vi "Video Stuff v11.vi"() -> ()   [LabVIEW 2009]
uses:
  <vilib>/userDefined/High Color/IMAQdx.ctl
  <vilib>/vision/NI_Vision_Development_Module.lvlib
  <vilib>/vision/driver/NI_Vision_Acquisition_Software.lvlib
panel:
  in  "Tab Control":enum32{"RGB", "RGB Adaptive", "Raphael", "Dan"}(tab)
  in  "Red Range":cluster{"Lower value":i32, "Upper value":i32}={"Lower value"=33, "Upper value"=255}
  in  "Green Range":cluster{"Lower value":i32, "Upper value":i32}={"Lower value"=0, "Upper value"=255}
  in  "Blue Range":cluster{"Lower value":i32, "Upper value":i32}={"Lower value"=0, "Upper value"=255}
  in  "Blue Scalar":sgl=3.3000002
  in  "Green Scalar":sgl=3.0
  in  "Red Scalar":sgl=4.0
  in  "Threshold Limits":cluster{"Lower value":sgl, "Upper value":sgl}={"Lower value"=0.0, "Upper value"=255.0} {"Upper value" format="%.2f"; "Lower value" format="%.2f"}
  out "Threshold Range Out":cluster{"Lower value":sgl, "Upper value":sgl}={"Lower value"=139.0, "Upper value"=255.0} {"Upper value" format="%.2f"; "Lower value" format="%.2f"}
  out "Number of Particles":i32=3
  in  "Selection Values":T2(array[cluster])=[{"Measurement Parameter"=35, "Range Lower Value"=100.0, "Range Upper Value"=10000.0, "Range"=FALSE, "Measurement Type"=FALSE}] {"Measurement Parameter" items=["Center of Mass X", "Center of Mass Y", "First Pixel X", "First Pixel Y", "Bounding Rect Left", "Bounding Rect Top", "Bounding Rect Right", "Bounding Rect Bottom", "Max Feret Diameter Start X", "Max Feret Diameter Start Y", "Max Feret Diameter End X", "Max Feret Diameter End Y", "Max Horiz. Segment Length Left", "Max Horiz. Segment Length Right", "Max Horiz. Segment Length Row", "-", "Bounding Rect Width", "Bounding Rect Height", "Bounding Rect Diagonal", "Perimeter", "Convex Hull Perimeter", "Holes' Perimeter", "Max Feret Diameter", "Equivalent Ellipse Major Axis", "Equivalent Ellipse Minor Axis", "Equivalent Ellipse Minor Axis (Feret)", "Equivalent Rect Long Side", "Equivalent Rect Short Side", "Equivalent Rect Diagonal", "Equivalent Rect Short Side (Feret)", "Average Horiz. Segment Length", "Average Vert. Segment Length", "Hydraulic Radius", "Waddel Disk Diameter", "-", "Area", "Holes' Area", "Particle & Holes' Area", "Convex Hull Area", "Image Area", "-", "Number of Holes", "Number of Horiz. Segments", "Number of Vert. Segments", "-", "Orientation", "Max Feret Diameter Orientation", "-", "% Area/Image Area", "% Area/(Particle & Holes' Area)", "Ratio of Equivalent Ellipse Axes", "Ratio of Equivalent Rect Sides", "-", "Elongation Factor", "Compactness Factor", "Heywood Circularity Factor", "Type Factor", "-", "Sum X", "Sum Y", "Sum XX", "Sum XY", "Sum YY", "Sum XXX", "Sum XXY", "Sum XYY", "Sum YYY", "-", "Moment of Inertia XX", "Moment of Inertia XY", "Moment of Inertia YY", "Moment of Inertia XXX", "Moment of Inertia XXY", "Moment of Inertia XYY", "Moment of Inertia YYY", "Norm. Moment of Inertia XX", "Norm. Moment of Inertia XY", "Norm. Moment of Inertia YY", "Norm. Moment of Inertia XXX", "Norm. Moment of Inertia XXY", "Norm. Moment of Inertia XYY", "Norm. Moment of Inertia YYY", "Hu Moment 1", "Hu Moment 2", "Hu Moment 3", "Hu Moment 4", "Hu Moment 5", "Hu Moment 6", "Hu Moment 7"]}
  in  "Filter Select":T3(radio)
  in  "bin 1    bin 2":bool
  in  "Select Filter":enum16{"RGB", "RGB Adaptive", "Raphael", "Dan"}(ring)=enum."RGB Adaptive"
  out "Live Video 2":T4(plugin-control)
  in  "Y Min":i32=2
  in  "Y Max":i32=13
  in  "X min":i32=2
  in  "X max":i32=15
  in  "Desired X Resolution":i32=640
  in  "LineFilterSelect":bool=TRUE
  out "Hough Intensity Graph":i32[][](graph)
  out "Angle 2":i32=25
  out "X Intercept 2":i32=-500
  in  "Hough Skip":i32=1
  out "Waypoint":cluster{i32, i32}={132, 5}
  in  "WP_DisplaySize/2":i32
  out "Filter Binary 2":T4(plugin-control)
  in  "Offset scale":dbl=1.51
  in  "Y":i32=1741
  in  "X":i32=777
  out "Real World Coordinates":cluster{"X":sgl, "Y":sgl}={"X"=76.907585, "Y"=411.85178} {"Y" format="%.2f"; "X" format="%.2f"}
  in  "Interpolation Type":u32(ring)=1 items=["Zero Order", "Bi-Linear", "Quadratic", "Cubic Spline"]
  in  "X Resolution":i32=640
  in  "Numeric":i32=21
  out "Occupancy Grid Square Size":dbl=5.022463525777591
  in  "LIDAR/Wheel Position Offset (in.)":dbl=60.0
  out "\"Obstickles\" y":dbl[](array[numeric])=[303.34102199907545, 303.34102199907545, 303.34102199907545, 303.34102199907545, 303.34102199907545, 295.75710207515135, 295.75710207515135, 295.75710207515135, 295.75710207515135, 295.75710207515135, 295.75710207515135, 295.75710207515135, 295.75710207515135, 295.75710207515135, 295.75710207515135, 295.75710207515135, 295.75710207515135, 295.75710207515135, 295.75710207515135, 288.1731821512272, 288.1731821512272, 288.1731821512272, 288.1731821512272, 288.1731821512272, 288.1731821512272, 288.1731821512272, 288.1731821512272, 288.1731821512272, 288.1731821512272, 288.1731821512272, 288.1731821512272, 288.1731821512272, 288.1731821512272, 288.1731821512272, 280.58926222730304, 280.58926222730304, 280.58926222730304, 280.58926222730304, 280.58926222730304, 280.58926222730304, 280.58926222730304, 280.58926222730304, 280.58926222730304, 280.58926222730304, 280.58926222730304, 280.58926222730304, 280.58926222730304, 280.58926222730304, 280.58926222730304, 280.58926222730304, 273.0053423033788, 273.0053423033788, 273.0053423033788, 273.0053423033788, 273.0053423033788, 273.0053423033788, 273.0053423033788, 273.0053423033788, 273.0053423033788, 273.0053423033788, 273.0053423033788, 273.0053423033788, 273.0053423033788, 273.0053423033788, 273.0053423033788, 273.0053423033788, 273.0053423033788, 265.4214223794547, 265.4214223794547, 265.4214223794547, 265.4214223794547, 265.4214223794547, 265.4214223794547, 265.4214223794547, 265.4214223794547, 265.4214223794547, 265.4214223794547, 265.4214223794547, 265.4214223794547, 265.4214223794547, 257.8375024555305, 257.8375024555305, 257.8375024555305, 257.8375024555305, 257.8375024555305, 257.8375024555305, 257.8375024555305, 257.8375024555305, 257.8375024555305, 257.8375024555305, 250.25358253160636, 250.25358253160636, 250.25358253160636, 250.25358253160636, 250.25358253160636, 250.25358253160636, 250.25358253160636, 250.25358253160636, 250.25358253160636, 250.25358253160636, 250.25358253160636, 242.6696626076822, 242.6696626076822, 242.6696626076822, 242.6696626076822, 242.6696626076822, 242.6696626076822, 242.6696626076822, 242.6696626076822, 235.085742683758, 235.085742683758, 235.085742683758, 235.085742683758, 235.085742683758, 235.085742683758, 227.50182275983389, 227.50182275983389, 227.50182275983389, 219.9179028359097, 219.9179028359097, 219.9179028359097, 219.9179028359097, 212.33398291198554, 212.33398291198554, 212.33398291198554, 212.33398291198554, 212.33398291198554, 212.33398291198554, 212.33398291198554, 212.33398291198554, 204.7500629880614, 204.7500629880614, 204.7500629880614, 204.7500629880614, 204.7500629880614, 189.58222314021305, 181.9983032162889, 174.41438329236473, 174.41438329236473, 166.83046336844058, 166.83046336844058, 159.2465434445164, 159.2465434445164, 159.2465434445164, 159.2465434445164, 159.2465434445164, 151.66262352059223, 151.66262352059223, 151.66262352059223, 144.07870359666808, 144.07870359666808, 144.07870359666808, 136.49478367274392, 136.49478367274392, 136.49478367274392, 136.49478367274392, 128.91086374881974, 128.91086374881974, 121.32694382489558, 113.74302390097142, 113.74302390097142, 106.15910397704727, 75.82342428135061]
  out "\"Obstickles\" x":dbl[](array[numeric])=[-83.4231191631658, -75.83919923924164, -68.25527931531747, -60.6713593913933, -53.087439467469146, -83.4231191631658, -75.83919923924164, -68.25527931531747, -60.6713593913933, -53.087439467469146, -30.33567969569665, -22.751759771772488, -15.167839847848326, -7.583919923924163, 0.0, 7.583919923924163, 15.167839847848326, 37.91959961962082, 45.503519543544975, -91.00703908708995, -83.4231191631658, -75.83919923924164, -68.25527931531747, -60.6713593913933, -53.087439467469146, -45.503519543544975, -30.33567969569665, -22.751759771772488, -7.583919923924163, 7.583919923924163, 22.751759771772488, 37.91959961962082, 45.503519543544975, 106.17487893493829, -98.59095901101412, -91.00703908708995, -83.4231191631658, -75.83919923924164, -68.25527931531747, -53.087439467469146, -45.503519543544975, -37.91959961962082, -22.751759771772488, 7.583919923924163, 15.167839847848326, 22.751759771772488, 30.33567969569665, 37.91959961962082, 75.83919923924164, 106.17487893493829, -106.17487893493829, -83.4231191631658, -75.83919923924164, -68.25527931531747, -60.6713593913933, -53.087439467469146, -37.91959961962082, -15.167839847848326, 7.583919923924163, 15.167839847848326, 22.751759771772488, 30.33567969569665, 37.91959961962082, 45.503519543544975, 53.087439467469146, 75.83919923924164, 98.59095901101412, -98.59095901101412, -83.4231191631658, -75.83919923924164, -68.25527931531747, 7.583919923924163, 15.167839847848326, 22.751759771772488, 30.33567969569665, 37.91959961962082, 45.503519543544975, 53.087439467469146, 75.83919923924164, 83.4231191631658, -45.503519543544975, -22.751759771772488, 7.583919923924163, 15.167839847848326, 22.751759771772488, 30.33567969569665, 37.91959961962082, 45.503519543544975, 60.6713593913933, 68.25527931531747, -37.91959961962082, -7.583919923924163, 0.0, 7.583919923924163, 15.167839847848326, 22.751759771772488, 30.33567969569665, 37.91959961962082, 45.503519543544975, 53.087439467469146, 60.6713593913933, -91.00703908708995, 7.583919923924163, 15.167839847848326, 22.751759771772488, 30.33567969569665, 37.91959961962082, 45.503519543544975, 53.087439467469146, -91.00703908708995, -7.583919923924163, 7.583919923924163, 15.167839847848326, 22.751759771772488, 37.91959961962082, -91.00703908708995, 7.583919923924163, 37.91959961962082, -22.751759771772488, 0.0, 22.751759771772488, 30.33567969569665, -15.167839847848326, 0.0, 7.583919923924163, 15.167839847848326, 22.751759771772488, 30.33567969569665, 53.087439467469146, 68.25527931531747, -30.33567969569665, 0.0, 22.751759771772488, 30.33567969569665, 45.503519543544975, 22.751759771772488, 30.33567969569665, 30.33567969569665, 60.6713593913933, -22.751759771772488, 30.33567969569665, -45.503519543544975, -22.751759771772488, 0.0, 30.33567969569665, 37.91959961962082, 22.751759771772488, 37.91959961962082, 45.503519543544975, 22.751759771772488, 45.503519543544975, 53.087439467469146, 0.0, 15.167839847848326, 22.751759771772488, 53.087439467469146, -15.167839847848326, 53.087439467469146, 60.6713593913933, 22.751759771772488, 68.25527931531747, 75.83919923924164, 15.167839847848326]
  out "Small":T4(plugin-control)
  in  "Horizontal Resolution of Small Image":i32=50
  out "Super Filter":T4(plugin-control)
  in  "Color Mode":u16(ring) items=["RGB", "HSL", "HSV", "HSI"]
  in  "stop":bool
  out "Calibrated Image":T4(plugin-control)
  out "Buffer Number":u32=946
  out "Live Video":T4(plugin-control)
  in  "Video Modes":i32(listbox)=20
  in  "Camera Name":T5="cam3"
  in  "Calibration File Path":path=path "C:/Documents and Settings/ekolker/My Documents/OGRE/vision/shoopCal.png"
  out "Top Image":T4(plugin-control) caption="Calibration Template"
  # "Line Width Paramaters"
  # "Indoor\nLower:\n   YUV?\n  150, 180, 20\n   RGB?\n  240, 240, 240"
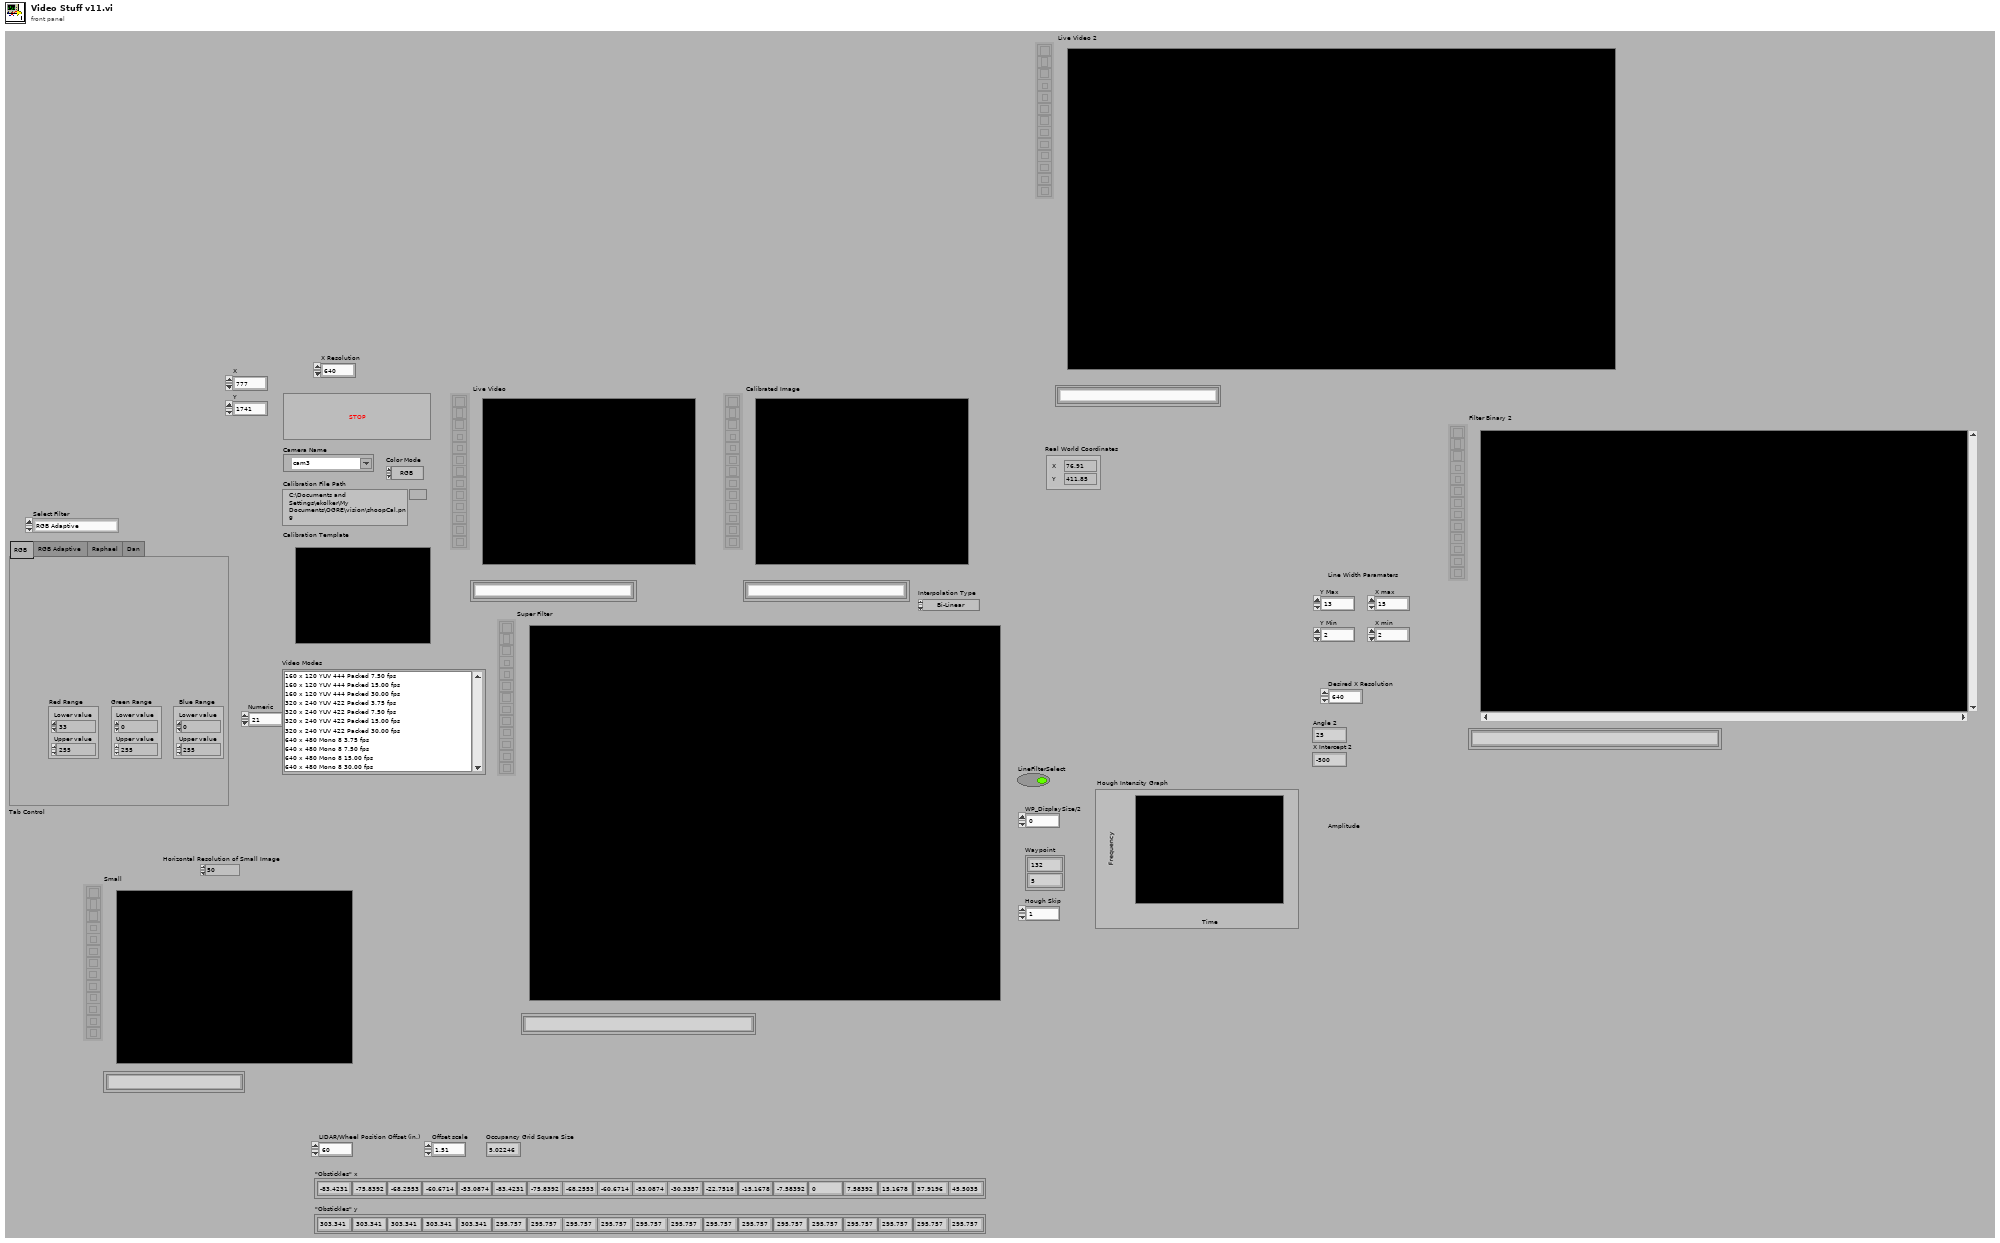
[diagram p1: front panel]
types:
  T1 = typedef "Particle Parameters" = i32
  T2 = cluster{"Measurement Parameter":T1, "Range Lower Value":dbl, "Range Upper Value":dbl, "Range":bool, "Measurement Type":bool}[]
  T3 = enum32{"RGB", "HSL", "RGB Adaptive", "HSL Adaptive", "ANN"}
  T4 = typedef "IMAQ Image.ctl" = refnum<image>
  T5 = typedef "IMAQdx.ctl" = refnum<k21>
  T6 = typedef "Image Type" = u32
  T7 = cluster{"X Step":sgl, "Y Step":sgl, "Unit":u32, "Threshold Range":cluster{"Lower value":sgl, "Upper value":sgl}}
  T8 = cluster{"Distortion":u32, "Corrected Image Scaling":u32, "Corrected Image Learn ROI":u32, "Learn Error Map?":bool, "Learn Correction Table?":bool}
  T9 = cluster{cluster{sgl, sgl}, "Angle Relative to Horizontal (deg)":sgl, "Axis Reference":u32}
  T10 = cluster{"Left":i32, "Top":i32, "Right":i32, "Bottom":i32}
  T11 = cluster{"histogram":u32[], "Minimal Value":sgl, "Maximal Value":sgl, "Starting Value":sgl, "Interval Width":sgl, "Mean Value":sgl, "Standard  Variation":sgl, "Area (pixels)":i32}
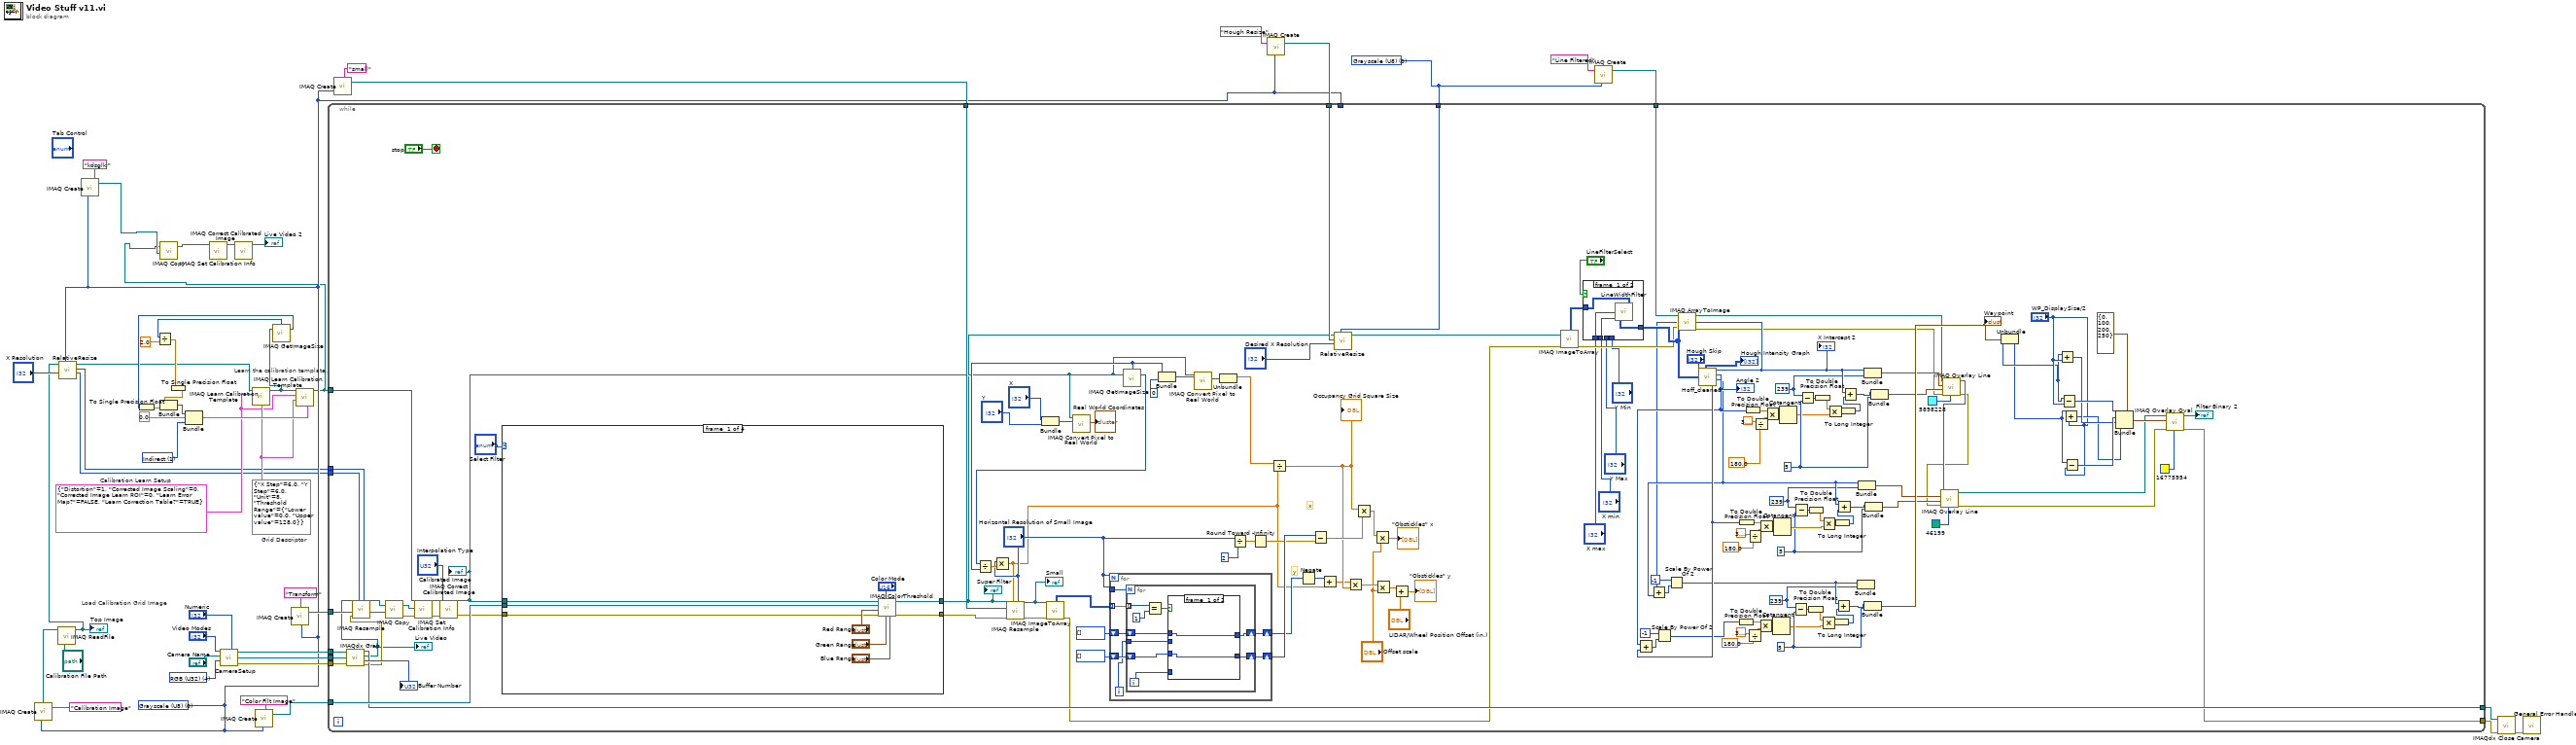
[diagram p0: block diagram]
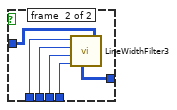
[diagram p2: hidden frame]
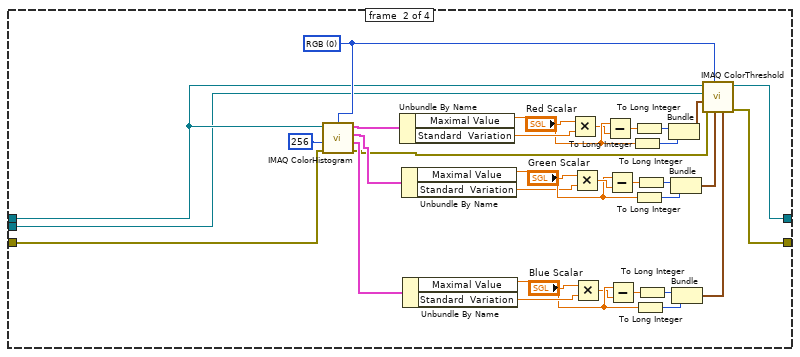
[diagram p3: hidden frame]
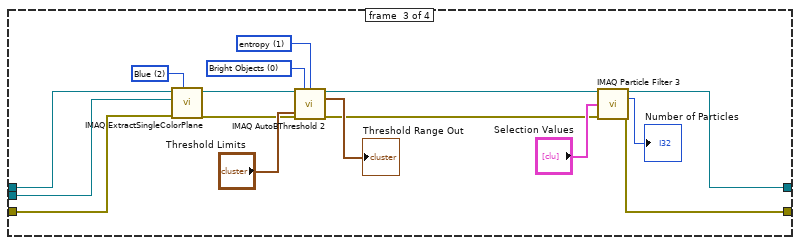
[diagram p4: hidden frame]
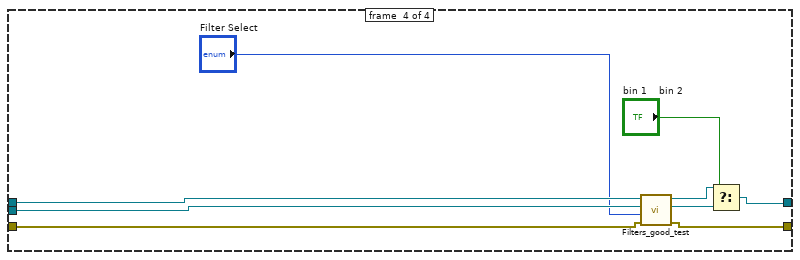
[diagram p5: hidden frame]
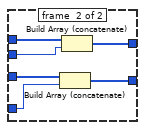
[diagram p6: hidden frame]
diagram:
  w1 = T6 0 items=["Grayscale (U8)", "Grayscale (I16)", "Grayscale (SGL)", "Complex (CSG)", "RGB (U32)", "HSL (U32)", "RGB (U64)", "Grayscale (U16)"] ("Image Type")
  w12 = T6 4 items=["Grayscale (U8)", "Grayscale (I16)", "Grayscale (SGL)", "Complex (CSG)", "RGB (U32)", "HSL (U32)", "RGB (U64)", "Grayscale (U16)"] ("Image Type")
  w31 = u32 1 items=["Direct", "Indirect"] ("Axis Reference")
  w9 = T6 0 items=["Grayscale (U8)", "Grayscale (I16)", "Grayscale (SGL)", "Complex (CSG)", "RGB (U32)", "HSL (U32)", "RGB (U64)", "Grayscale (U16)"] ("Image Type")
  w21 = T7 {"X Step"=6.0, "Y Step"=6.0, "Unit"=8, "Threshold Range"={"Lower value"=0.0, "Upper value"=128.0}}  # Grid Descriptor
  w20 = T8 {"Distortion"=1, "Corrected Image Scaling"=0, "Corrected Image Learn ROI"=0, "Learn Error Map?"=FALSE, "Learn Correction Table?"=TRUE}  # Calibration Learn Setup
  # "Load Calibration Grid Image"
  # "Learn the calibration template."
  n1 = call "IMAQ Create"("Image Name"="Calibration Image", "Image Type"=w9) -> ("New Image"=w39:T4)  [unwired: 2 in, 2 out]
  n2 = call "IMAQ ReadFile"("File Path"="Calibration File Path", "Image"=w39) -> ("Image Out"=w15:T4)  [unwired: 3 in, 6 out]
  "Top Image" <- w15
  n3 = call "RelativeResize.vi"("Image Type"=w9, "Desired X Resolution"="X Resolution", "Image"=w15) -> ("Y Resolution"=w5:i32, "X Resolution"=w4:i32, "Image Dst Out"=w16:T4)  [unwired: 3 in, 1 out]
  n4 = call "IMAQ Create"("Image Name"="kdsglk;", "Image Type"=w9) -> ("New Image"=w3:T4)  [unwired: 2 in, 2 out]
  n5 = call "CameraSetup.vi"("Video Modes"="Video Modes", "Camera Name"="Camera Name", "Image Type"=w12, "Numeric"="Numeric") -> ("Session Out"=w42:T5, "New Image"=w41:T4, "error out"=w40:errorcluster)  [unwired: 2 in]
  n6 = call "IMAQ Learn Calibration Template"("Grid Descriptor"=w21, "Calibration Learn Setup"=w20, "Image"=w16) -> ("Calibrated Image"=w7:T4)  [unwired: 4 in, 4 out]
  n7 = call "IMAQ Create"("Image Name"="Color Filt Image", "Image Type"=w9) -> ("New Image"=w38:T4)  [unwired: 2 in, 2 out]
  n8 = call "IMAQ GetImageSize"("Image"=w7) -> ("Y Resolution"=w25:i32, "X Resolution"=w26:i32)  [unwired: 3 in, 1 out]
  n9 = To Single Precision Float(number=w25) -> (single precision float=w24:sgl)
  n10 = Divide(x=w26, y=2.0) -> (x/y=w23:dbl)
  n11 = To Single Precision Float(number=w23) -> (single precision float=w22:sgl)
  n12 = Bundle(w22, w24) -> (w29:cluster{sgl, sgl})  [unwired: 1 in]
  n13 = Bundle(w29, "Angle Relative to Horizontal (deg)"=sgl 0.0, "Axis Reference"=w31) -> (w28:T9)  [unwired: 1 in]
  n14 = call "IMAQ Create"("Image Name"="Transform", "Image Type"=w9) -> ("New Image"=w43:T4)  [unwired: 2 in, 2 out]
  n15 = call "IMAQ Learn Calibration Template"("Calibration Axis Info"=w28, "Grid Descriptor"=w21, "Calibration Learn Setup"=w20, "Image"=w7) -> ("Calibrated Image"=w2:T4)  [unwired: 3 in, 4 out]
  n16 = call "IMAQ Copy"("Image Dst"=w3, "Image Src"=w2) -> ("Image Dst Out"=w6:T4)  [unwired: 4 in, 1 out]
  n17 = call "IMAQ Set Calibration Info"("Image Src"=w6) -> ("Calibrated Image"=w11:T4)  [unwired: 3 in, 7 out]
  n18 = call "IMAQ Correct Calibrated Image"("Image Src"=w11) -> ("Corrected Image"=→"Live Video 2":T4)  [unwired: 6 in, 4 out]
  n19 = call "IMAQ Create"("Image Name"="small", "Image Type"=w9) -> ("New Image"=w36:T4)  [unwired: 2 in, 2 out]
  n20 = call "IMAQ Create"("Image Name"="Hough Resize", "Image Type"=w9) -> ("New Image"=w13:T4)  [unwired: 2 in, 2 out]
  n21 = call "IMAQ Create"("Image Name"="Line Filtered", "Image Type"=w1) -> ("New Image"=w18:T4)  [unwired: 2 in, 2 out]
  n22 = while {
    tunnel: w2 -> [w165]
    tunnel: w43 -> [w193]
    tunnel: w42 -> [w192]
    tunnel: w41 -> [w191]
    tunnel: w40 -> [w190]
    tunnel: w38 -> [w186]
    tunnel: w36 -> [w184]
    tunnel: [w182] -> w34
    tunnel: [w126] -> w33
    tunnel: w18 -> [w125]
    tunnel: w4 -> [w65]
    tunnel: w5 -> [w64]
    tunnel: w13 -> [w61]
    tunnel: w9 -> [_]
    tunnel: w1 -> [w60]
    stop <- "stop" stop-if-true
    w110 = 5 ("y")
    w109 = 239 ("y")
    w88 = 5 ("y")
    w89 = 239 ("y")
    w77 = 5 ("y")
    w76 = 239 ("y")
    # "y"
    # "x"
    n23 = call <vilib>:"IMAQdx Grab.vi"("error in"=w190, "Image In"=w191, "Session In"=w192) -> ("error out"=w168:errorcluster, "Buffer Number Out"=→"Buffer Number":u32, "Image Out"=w167:T4, "Session Out"=w182:T5)  [unwired: 1 in, 4 out]
    "Live Video" <- w167
    n24 = call "IMAQ Resample"("X Resolution"=w65, "Y Resolution"=w64, "error in (no error)"=w168, "Image Src"=w167) -> ("Image Dst Out"=w166:T4)  [unwired: 6 in, 1 out]
    n25 = call "IMAQ Copy"("Image Dst"=w193, "Image Src"=w166) -> ("error out"=w194:errorcluster, "Image Dst Out"=w197:T4)  [unwired: 4 in]
    n26 = call "IMAQ Set Calibration Info"("error in (no error)"=w194, "Image Dst"=w197, "Image Src"=w165) -> ("error out"=w195:errorcluster, "Calibrated Image"=w196:T4)  [unwired: 1 in, 6 out]
    n27 = call "IMAQ Correct Calibrated Image"("Interpolation Type"="Interpolation Type", "error in (no error)"=w195, "Image Src"=w196) -> ("error out"=w185:errorcluster, "Corrected Image"=w57:T4)  [unwired: 4 in, 3 out]
    "Calibrated Image" <- w57
    n28 = case shown="\"Raphael\"" "Select Filter" {
      tunnel: [w213 w218 w253 w276] -> w189
      tunnel: [w212 w221 w256 w273] -> w56
      tunnel: w186 -> [w211 w222 w262 w274]
      tunnel: w185 -> [w210 w220 w261 w277]
      tunnel: w57 -> [w209 w223 w263 w275]
      frame #0 {
        n29 = call "IMAQ ColorThreshold"("Blue or Luma or Val or Inten Range"="Blue Range", "Green or Sat Range"="Green Range", "Color Mode"="Color Mode", "error in (no error)"=w210, "Red or Hue Range"="Red Range", "Image Dst"=w211, "Image Src"=w209) -> ("error out"=w213:errorcluster, "Image Dst Out"=w212:T4)  [unwired: 3 in]
      }
      frame #1 {
        w251 = u16 0 items=["RGB", "HSL", "HSV", "HSI"] ("Color Mode")
        n30 = call "IMAQ ColorHistogram"("Color Mode"=w251, "Image Src"=w223, "Number of Classes"=256, "error in (no error)"=w220) -> ("Red or Hue or X or L* Histogram Report"=w250:T11, "Green or Sat or Y or a* Histogram Report"=w225:T11, "Blue or Luma or Val or Inten or Z or b* Histogram Report"=w224:T11, "error out"=w219:errorcluster)  [unwired: 2 in]
        n31 = Unbundle By Name(w250) -> ("Maximal Value"=w244:sgl, "Standard  Variation"=w246:sgl)
        n32 = Unbundle By Name(w225) -> ("Maximal Value"=w239:sgl, "Standard  Variation"=w237:sgl)
        n33 = Unbundle By Name(w224) -> ("Maximal Value"=w230:sgl, "Standard  Variation"=w232:sgl)
        n34 = Multiply(x="Red Scalar", y=w246) -> (x*y=w243:sgl)
        n35 = Multiply(x="Green Scalar", y=w237) -> (x*y=w240:sgl)
        n36 = Multiply(x="Blue Scalar", y=w232) -> (x*y=w229:sgl)
        n37 = Subtract(x=w244, y=w243) -> (x-y=w245:sgl)
        n38 = Subtract(x=w239, y=w240) -> (x-y=w238:sgl)
        n39 = Subtract(x=w230, y=w229) -> (x-y=w231:sgl)
        n40 = To Long Integer(number=w244) -> (32bit integer=w247:i32)
        n41 = To Long Integer(number=w245) -> (32bit integer=w248:i32)
        n42 = To Long Integer(number=w239) -> (32bit integer=w236:i32)
        n43 = To Long Integer(number=w230) -> (32bit integer=w233:i32)
        n44 = To Long Integer(number=w238) -> (32bit integer=w235:i32)
        n45 = To Long Integer(number=w231) -> (32bit integer=w234:i32)
        n46 = Bundle(w248, w247) -> (w249:cluster{i32, i32})  [unwired: 1 in]
        n47 = Bundle(w235, w236) -> (w227:cluster{i32, i32})  [unwired: 1 in]
        n48 = Bundle(w234, w233) -> (w226:cluster{i32, i32})  [unwired: 1 in]
        n49 = call "IMAQ ColorThreshold"("Blue or Luma or Val or Inten Range"=w226, "Green or Sat Range"=w227, "Color Mode"=w251, "error in (no error)"=w219, "Red or Hue Range"=w249, "Image Dst"=w222, "Image Src"=w223) -> ("error out"=w218:errorcluster, "Image Dst Out"=w221:T4)  [unwired: 3 in]
      }
      frame #2 {
        w258 = 1 items=["clustering", "entropy", "metric", "moments", "inter-class variance"] ("Method (clustering)")
        w259 = u32 0 items=["Bright Objects", "Dark Objects"] ("Look For (Bright Objects)")
        w260 = 2 items=["Red", "Green", "Blue", "Hue", "Saturation", "Luminance", "Value", "Intensity"] ("Color Plane")
        n50 = call "IMAQ ExtractSingleColorPlane"("Color Plane"=w260, "error in (no error)"=w261, "Image Dst"=w262, "Image Src"=w263) -> ("error out"=w255:errorcluster, "Image Dst Out"=w268:T4)  [unwired: 6 in]
        n51 = call "IMAQ AutoBThreshold 2"("Image Src"=w268, "Look For (Bright Objects)"=w259, "Method (clustering)"=w258, "error in (no error)"=w255, "Threshold Limits"="Threshold Limits") -> ("Image Dst Out"=w265:T4, "Threshold Range Out"=→"Threshold Range Out":cluster{"Lower value":sgl, "Upper value":sgl}, "error out"=w254:errorcluster)  [unwired: 8 in]
        n52 = call "IMAQ Particle Filter 3"("Image Src"=w265, "Selection Values"="Selection Values", "error in (no error)"=w254) -> ("Image Dst Out"=w256:T4, "Number of Particles"=→"Number of Particles":i32, "error out"=w253:errorcluster)  [unwired: 10 in]
      }
      frame #3 {
        n53 = call "Filters_good_test.vi"("error in"=w277, "Filter Select"="Filter Select", "Filter"=w274, "Input"=w275) -> ("error out"=w276:errorcluster, "Filter Binary"=w272:T4, "Filter Binary 2"=w271:T4)  [unwired: 5 in]
        n54 = Select(t=w271, s="bin 1    bin 2", f=w272) -> (s? t:f=w273:T4)
      }
    }
    "Super Filter" <- w56
    n55 = Bundle("X"="X", "Y"="Y") -> (w161:cluster{"X":i32, "Y":i32})  [unwired: 1 in]
    n56 = call "IMAQ Convert Pixel to Real World"("Pixel Coordinates"=w161, "Calibrated Image"=w57) -> ("Real World Coordinates"=→"Real World Coordinates":cluster{"X":sgl, "Y":sgl})  [unwired: 4 in, 5 out]
    n57 = call "IMAQ GetImageSize"("Image"=w57) -> ("Y Resolution"=w153:i32, "X Resolution"=w152:i32)  [unwired: 3 in, 1 out]
    n58 = Divide(x=w153, y=w152) -> (x/y=w155:dbl)
    n59 = Multiply(x="Horizontal Resolution of Small Image", y=w155) -> (x*y=w146:dbl)
    n60 = call "IMAQ Resample"("X Resolution"="Horizontal Resolution of Small Image", "Y Resolution"=w146, "error in (no error)"=w189, "Image Dst"=w184, "Image Src"=w56) -> ("error out"=w188:errorcluster, "Image Dst Out"=w129:T4)  [unwired: 5 in]
    "Small" <- w129
    n61 = call "IMAQ ImageToArray"("error in (no error)"=w188, "Image"=w129) -> ("error out"=w127:errorcluster, "Image Pixels (U8)"=w179:u8[][])  [unwired: 2 in, 3 out]
    n62 = for {
      N: "Horizontal Resolution of Small Image" -> [_]
      tunnel: "Horizontal Resolution of Small Image" -> [w284]
      tunnel: w179 -> [w283] mode=indexing
      shift-right: [w282] -> w178
      shift-left: i32[] [] -> [w281]
      shift-right: [w279] -> w171
      shift-left: i32[] [] -> [w278]
      i -> [w280]
      n63 = for {
        N: w284 -> [_]
        tunnel: w283 -> [w293] mode=indexing
        shift-right: [w289] -> w282
        shift-left: w281 -> [w288]
        tunnel: w280 -> [w287]
        shift-right: [w286] -> w279
        shift-left: w278 -> [w285]
        i -> [w291]
        n64 = Equal?(x=w293, y=u8 1) -> (x = y?=w290:bool)
        n65 = case shown="False" w290 {
          tunnel: w291 -> [_ w301]
          tunnel: [w294 w300] -> w289
          tunnel: w288 -> [w294 w299]
          tunnel: w287 -> [_ w298]
          tunnel: [w295 w297] -> w286
          tunnel: w285 -> [w295 w296]
          frame #0 {
          }
          frame #1 {
            n66 = Build Array (concatenate)(w299, w301) -> (w300:i32[])
            n67 = Build Array (concatenate)(w296, w298) -> (w297:i32[])
          }
        }
      }
    }
    n68 = Bundle("X Resolution"=w152, 0) -> (w163:cluster{"X Resolution":i32, i32})  [unwired: 1 in]
    n69 = call "IMAQ Convert Pixel to Real World"("Pixel Coordinates"=w163, "Calibrated Image"=w57) -> ("Real World Coordinates"=w157:cluster{"X":sgl, "Y":sgl})  [unwired: 4 in, 5 out]
    n70 = Unbundle(w157) -> ("X"=w156:sgl)  [unwired: 1 out]
    n71 = Divide(x="Horizontal Resolution of Small Image", y=2) -> (x/y=w170:dbl)
    n72 = Round Toward -Infinity(1:w170) -> (0:w169:dbl)
    n73 = Divide(x=w156, y=w146) -> (x/y=w176:dbl)
    "Occupancy Grid Square Size" <- w176
    n74 = Negate(x=w171) -> (-x=w172:i32[])
    n75 = Subtract(x=w178, y=w169) -> (x-y=w177:dbl[])
    n76 = Add(x=w172, y=w146) -> (x+y=w175:dbl[])
    n77 = call "RelativeResize.vi"("Image Type"=w60, "Desired X Resolution"="Desired X Resolution", "Image Dst"=w61, "Image"=w56) -> ("Image Dst Out"=w63:T4)  [unwired: 2 in, 3 out]
    n78 = Multiply(x=w175, y=w176) -> (x*y=w151:dbl[])
    n79 = Multiply(x=w176, y=w177) -> (x*y=w149:dbl[])
    n80 = Multiply(x=w149, y="Offset scale") -> (x*y=→"\"Obstickles\" x":dbl[])
    n81 = Multiply(x=w151, y="Offset scale") -> (x*y=w150:dbl[])
    n82 = Add(x=w150, y="LIDAR/Wheel Position Offset (in.)") -> (x+y=→"\"Obstickles\" y":dbl[])
    n83 = call "IMAQ ImageToArray"("error in (no error)"=w127, "Image"=w63) -> ("error out"=w128:errorcluster, "Image Pixels (U8)"=w130:u8[][])  [unwired: 2 in, 3 out]
    n84 = case shown="False" "LineFilterSelect" {
      tunnel: w130 -> [w200 w207]
      tunnel: [w202 w208] -> w133
      tunnel: "X max" -> [w201 w206]
      tunnel: "X min" -> [w199 w205]
      tunnel: "Y Max" -> [_ w204]
      tunnel: "Y Min" -> [_ w203]
      frame #0 {
        n85 = call "LineWidthFilter.vi"("Image Pixels (U8) 2"=w200, "X Min"=w199, "X max"=w201) -> ("Image Pixels (U8)"=w202:u8[][])
      }
      frame #1 {
        n86 = call "LineWidthFilter3.vi"("X max"=w206, "X min"=w205, "Y Max"=w204, "Y Min"=w203, "Image Pixels (U8) 2"=w207) -> ("Image Pixels (U8)"=w208:u8[][])
      }
    }
    n87 = call "IMAQ ArrayToImage"("error in (no error)"=w128, "Image Pixels (U8)"=w133, "Image"=w125) -> ("error out"=w66:errorcluster, "Image Out"=w59:T4)  [unwired: 7 in]
    n88 = call "Hoff_cleaned.vi"("Skip-1"="Hough Skip", "Image Pixels (U8)"=w133) -> ("3 times averaged"=→"Hough Intensity Graph":i32[][], "X Intercept"=w121:i32, "Angle"=w123:i32, "X Intercept 2"=w122:i32, "Angle 2"=w124:i32)  [unwired: 2 in]
    "Angle 2" <- w123
    "X Intercept 2" <- w121
    n89 = Add(x=w123, y=w124) -> (x+y=w120:i32)
    n90 = Add(x=w121, y=w122) -> (x+y=w119:i32)
    n91 = Scale By Power Of 2(n=i16 -1, x=w120) -> (x*2^n=w116:i32)
    n92 = Scale By Power Of 2(n=i16 -1, x=w119) -> (x*2^n=w118:i32)
    n93 = To Double Precision Float(number=w116) -> (double precision float=w104:dbl)
    n94 = To Double Precision Float(number=w124) -> (double precision float=w94:dbl)
    n95 = To Double Precision Float(number=w123) -> (double precision float=w71:dbl)
    n96 = Divide(x=3.141592653589793, y=180.0) -> (x/y=w105:dbl)
    n97 = Divide(x=3.141592653589793, y=180.0) -> (x/y=w93:dbl)
    n98 = Divide(x=3.141592653589793, y=180.0) -> (x/y=w72:dbl)
    n99 = Multiply(x=w104, y=w105) -> (x*y=w106:dbl)
    n100 = Multiply(x=w94, y=w93) -> (x*y=w92:dbl)
    n101 = Multiply(x=w71, y=w72) -> (x*y=w73:dbl)
    n102 = Cotangent(1:w106) -> (0:w107:dbl)
    n103 = Cotangent(1:w92) -> (0:w91:dbl)
    n104 = Cotangent(1:w73) -> (0:w74:dbl)
    n105 = Subtract(x=w109, y=w110) -> (x-y=w111:i32)
    n106 = Subtract(x=w89, y=w88) -> (x-y=w87:i32)
    n107 = Subtract(x=w76, y=w77) -> (x-y=w80:i32)
    n108 = To Double Precision Float(number=w111) -> (double precision float=w112:dbl)
    n109 = To Double Precision Float(number=w87) -> (double precision float=w86:dbl)
    n110 = To Double Precision Float(number=w80) -> (double precision float=w81:dbl)
    n111 = Multiply(x=w112, y=w107) -> (x*y=w113:dbl)
    n112 = Multiply(x=w86, y=w91) -> (x*y=w85:dbl)
    n113 = Multiply(x=w81, y=w74) -> (x*y=w82:dbl)
    n114 = To Long Integer(number=w113) -> (32bit integer=w114:i32)
    n115 = To Long Integer(number=w85) -> (32bit integer=w84:i32)
    n116 = Add(x=w118, y=w114) -> (x+y=w108:i32)
    n117 = Add(x=w122, y=w84) -> (x+y=w90:i32)
    n118 = To Long Integer(number=w82) -> (32bit integer=w83:i32)
    n119 = Add(x=w121, y=w83) -> (x+y=w75:i32)
    n120 = Bundle(w118, "y"=w109) -> ()  [unwired: 1 in, 1 out]
    n121 = Bundle("X Intercept 2"=w122, "y"=w89) -> (w99:cluster{"X Intercept 2":i32, "y":i32})  [unwired: 1 in]
    n122 = Bundle("X Intercept"=w121, "y"=w76) -> (w78:cluster{"X Intercept":i32, "y":i32})  [unwired: 1 in]
    n123 = Bundle(w108, "y"=w110) -> (w134:cluster{i32, "y":i32})  [unwired: 1 in]
    "Waypoint" <- w134
    n124 = Bundle(w90, "y"=w88) -> (w100:cluster{i32, "y":i32})  [unwired: 1 in]
    n125 = Bundle(w75, "y"=w77) -> (w79:cluster{i32, "y":i32})  [unwired: 1 in]
    n126 = call "IMAQ Overlay Line"("Color"=u32 5898228, "error in (no error)"=w66, "End Point"=w79, "Start Point"=w78, "Image"=w59) -> ("error out"=w51:errorcluster, "Image Out"=w101:T4)  [unwired: 5 in]
    n127 = call "IMAQ Overlay Line"("Color"=u32 46199, "error in (no error)"=w51, "End Point"=w100, "Start Point"=w99, "Image"=w101) -> ("error out"=w131:errorcluster, "Image Out"=w137:T4)  [unwired: 5 in]
    n128 = Unbundle(w134) -> (w136:i32, "y"=w135:i32)
    n129 = Add(x=w136, y="WP_DisplaySize/2") -> (x+y=w142:i32)
    n130 = Subtract(x=w136, y="WP_DisplaySize/2") -> (x-y=w144:i32)
    n131 = Add(x=w135, y="WP_DisplaySize/2") -> (x+y=w141:i32)
    n132 = Subtract(x=w135, y="WP_DisplaySize/2") -> (x-y=w143:i32)
    n133 = Bundle(cluster=T10 {"Left"=0, "Top"=100, "Right"=200, "Bottom"=250} ("Bounding Rectangle"), "Left"=w144, "Top"=w143, "Right"=w142, "Bottom"=w141) -> (w140:T10)
    n134 = call "IMAQ Overlay Oval"("Color"=u32 16775954, "error in (no error)"=w131, "Bounding Rectangle"=w140, "Image"=w137) -> ("error out"=w126:errorcluster, "Image Out"=→"Filter Binary 2":T4)  [unwired: 6 in]
  }
  n135 = call <vilib>:"IMAQdx Close Camera.vi"("error in"=w33, "Session In"=w34) -> ("error out"=w35:errorcluster)  [unwired: 9 out]
  n136 = call <vilib>:"General Error Handler.vi"("error in (no error)"=w35) -> ()  [unwired: 1 in, 14 out]
